vi "fpga_main.vi"() -> ()   [LabVIEW 2019]
uses:
  <vilib>/Platform/TimedLoop/XDataNode/timing_clust.ctl
  <vilib>/Platform/TimedLoop/XDataNode/nitl_modes.ctl
  <vilib>/Platform/TimedLoop/XDataNode/wakeup.ctl
  <vilib>/rvi/Emulation/niFpgaSctlEmulationGetInTimedLoop.vi
  <vilib>/rvi/Emulation/niFpgaEmulationReportErrorSimple.vi
  <vilib>/rvi/Emulation/niFpgaGetClockAttributes.vi
  <vilib>/rvi/Emulation/niFpgaCriticalErrorInLSC.vi
  <vilib>/rvi/eio/common/nirviEmuTemplateMethod_errors.vi
  <vilib>/rvi/Memory/Memory_Emulation/nirvimemoryFastEmulation.vi
  <vilib>/rvi/Memory/Memory_Emulation/nirvimemoryEmulation.vi
  <vilib>/rvi/Emulation/niFpgaEmulationIsFPGAContextNoSignature.vi
  <vilib>/rvi/DataTransferAndStorage/Container/Common/niFpgaContainerGetUniqueNameForEmu.vi
  <vilib>/rvi/Emulation/niFpgaProcessEmulError.vi
  <vilib>/rvi/errors/nirviReportUnexpectedCaseInternalError (U32).vi
  <vilib>/rvi/interface/RandomDataEmulation/niFpgaRandomDataHandleErrors.vi
  <vilib>/Platform/TimedLoop/XDataNode/XDataNode.xnode
  <vilib>/eio/EIONode/EIONode.xnode
  <vilib>/rvi/DataTransferAndStorage/Container/XNode/niFpgaContainer.xnode
  <vilib>/rvi/interface/RandomDataEmulation/nirviRandomDataFpgaReadWriteTemplate.vi
  <vilib>/Platform/TimedLoop/XDataNode/XDNodeRunTimeDep.lvlib
panel:
  in  "prog ncmd":u32
  in  "default out":u8
  in  "software trig":bool=TRUE
  in  "persistent trig":bool=TRUE
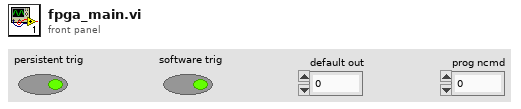
[diagram p1: front panel]
types:
  T1 = cluster{"state":enum8{"exec", "prog"}, "address":u32, "tic":u64, "init?":bool}
  T2 = typedef "XDNodeRunTimeDep.lvlib/timing_clust.ctl" = cluster{"Expected End [f-1]":u64, "Actual End [f-1]":u64, "Finished Late? [f-1]":bool, "Expected End [i-1]":u64, "Actual End [i-1]":u64, "Finished Late? [i-1]":bool, "Expected Start [i]":u64, "Actual Start [i]":u64, "Expected Start [f]":u64, "Actual Start [f]":u64, "Source Name":string, "Structure Name":string, "Period":i64, "Deadline":i64, "Offset":i64, "Start":i64, "Priority":i32, "Timeout":i32, "Mode":T3, "Wakeup Reason":T4, "Error":errorcluster, "Source Type":string, "Secondary Source Type":string, "Global End Time":u64, "Global Start Time":u64, "Frame Duration":u64, "Iteration Duration":u64, "Assigned CPU":i32, "I/O Scan Engine Mode":u32}
  T3 = typedef "XDNodeRunTimeDep.lvlib/nitl_modes.ctl" = enum32{"No Change", "Process missed periods, maintain original phase", "Discard missed periods, maintain original phase", "Process missed periods, ignore original phase", "Discard missed periods, ignore original phase"}
  T4 = typedef "XDNodeRunTimeDep.lvlib/wakeup.ctl" = enum32{"Normal", "Aborted", "Asynchronous wakeup", "Timing source error", "Timed loop error", "Timeout"}
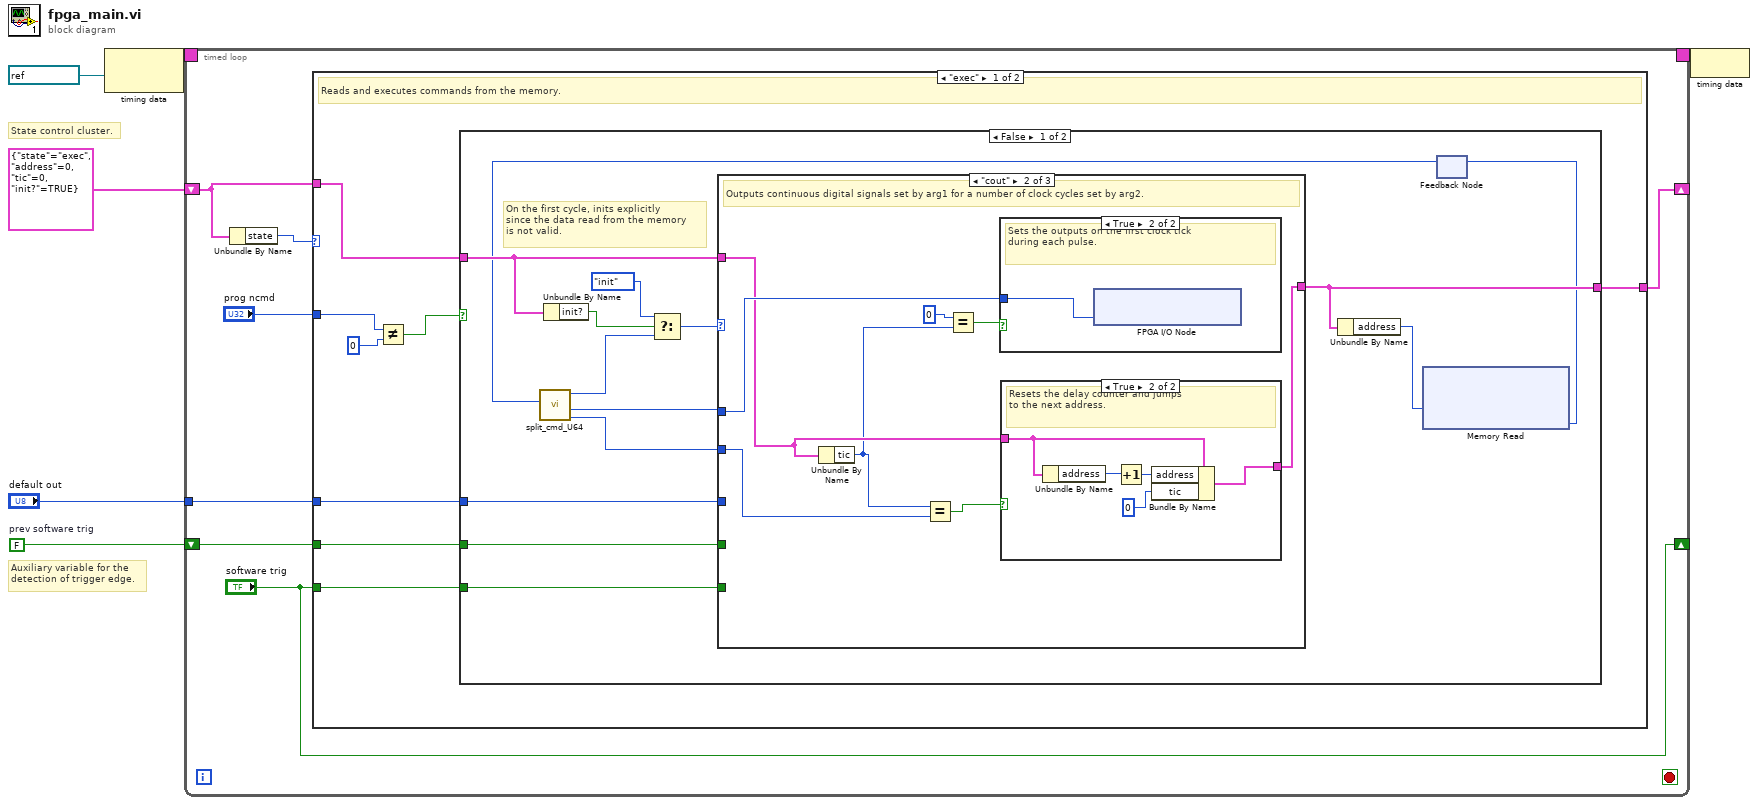
[diagram p0: block diagram]
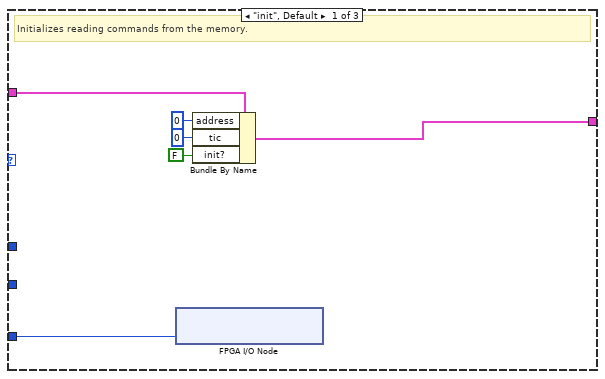
[diagram p2: hidden frame]
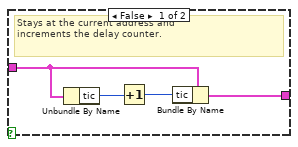
[diagram p4: hidden frame]
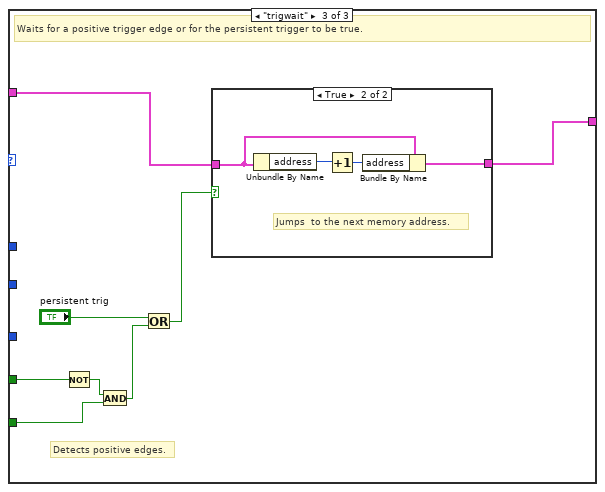
[diagram p5: hidden frame]
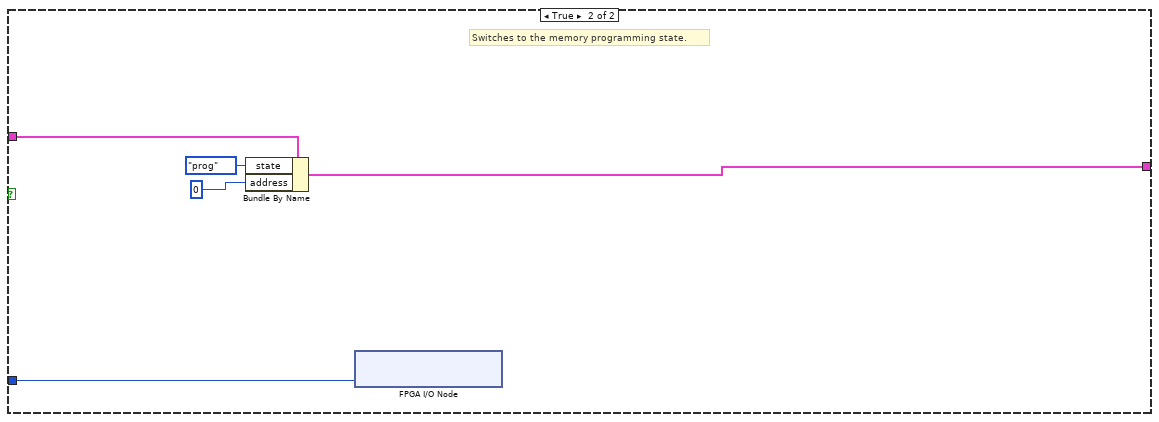
[diagram p7: hidden frame]
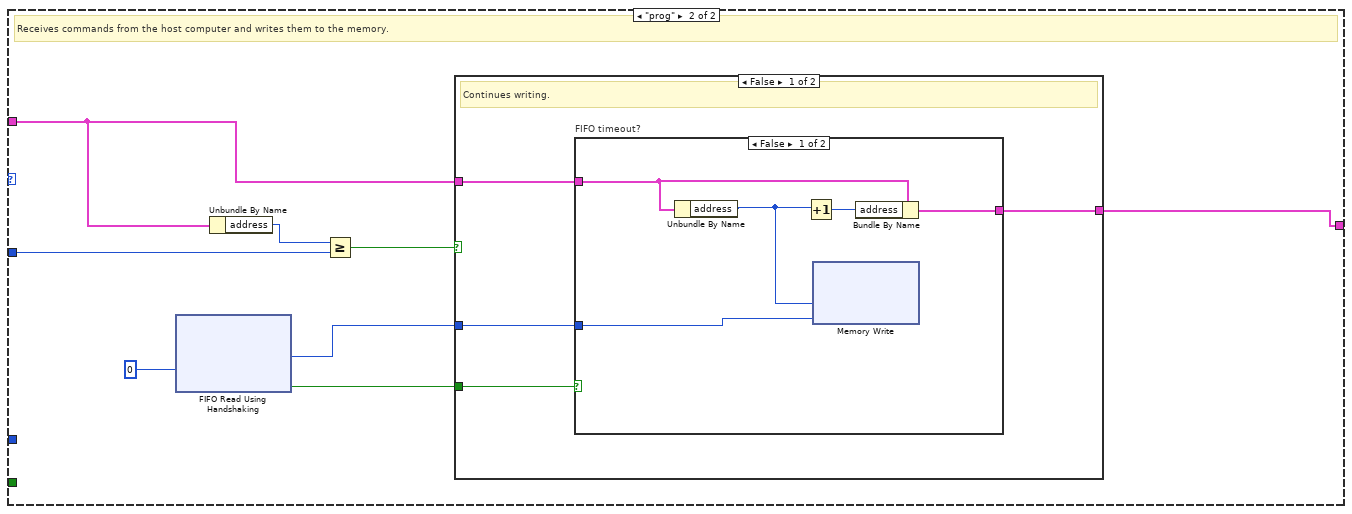
[diagram p8: hidden frame]
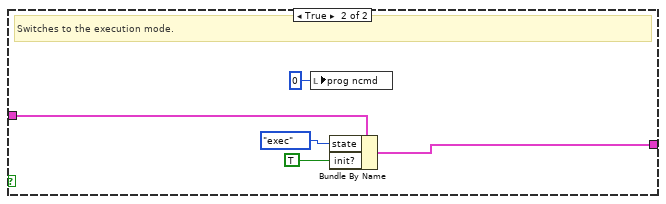
[diagram p10: hidden frame]
diagram:
  w1 = FALSE  # prev software trig
  # "Auxiliary variable for the \ndetection of trigger edge."
  # "State control cluster."
  n1 = node-c288(refnum<k21> "100MHz" ("Source Name")) -> (w6:T2)
  n2 = timed-loop {
    timing: w6 -> [_]
    timing-out: [_] -> w5
    shift-right: [w11] -> _
    shift-left: T1 {"state"=enum."exec", "address"=0, "tic"=0, "init?"=TRUE} -> [w12]
    tunnel: "default out" -> [w10]
    shift-right: ["software trig"] -> _
    shift-left: w1 -> [w9]
    stop <- _ stop-if-true
    n3 = Unbundle By Name(w12) -> ("state"=w13:enum8{"exec", "prog"})
    n4 = case shown="\"exec\"" w13 {
      tunnel: w12 -> [w21 w83]
      tunnel: [w20 w85] -> w11
      tunnel: w10 -> [w17 _]
      tunnel: w9 -> [w16 _]
      tunnel: "software trig" -> [w15 _]
      tunnel: "prog ncmd" -> [w14 w82]
      frame "exec" {
        # "Reads and executes commands from the memory."
        n5 = Not Equal?(x=w14, y=u32 0 ("x")) -> (x != y?=w19:bool)
        n6 = case shown="False" w19 {
          tunnel: w21 -> [w27 w77]
          tunnel: [w34 w76] -> w20
          tunnel: w17 -> [w35 w74]
          tunnel: w16 -> [w32 _]
          tunnel: w15 -> [w31 _]
          frame False {
            # "On the first cycle, inits explicitly \nsince the data read from the memory \nis not valid."
            n7 = Unbundle By Name(w27) -> ("init?"=w26:bool)
            n8 = feedback #1() -> (w25:u64)  [unwired: 1 in]
            n9 = call "split_cmd_U64.vi"("command"=w25) -> ("arg2"=w22:u64, "arg1"=w23:u8, "name"=w24:enum8{"init", "cout", "trigwait"})  [unwired: 7 in]
            n10 = Select(t=enum8{"init", "cout", "trigwait"}."init", s=w26, f=w24) -> (s? t:f=w29:enum8{"init", "cout", "trigwait"})
            n11 = case shown="\"cout\"" w29 {
              tunnel: w35 -> [w41 _ _]
              tunnel: [w38 w44 w65] -> w34
              tunnel: w27 -> [w40 w43 w66]
              tunnel: w23 -> [_ w46 _]
              tunnel: w32 -> [_ _ w63]
              tunnel: w31 -> [_ _ w61]
              tunnel: w22 -> [_ w45 _]
              frame "init", Default {
                # "Initializes reading commands from the memory."
                n12 = xnode "FPGA I/O Node"("ConnectorA/DIO7:0"=w41) -> ()  [unwired: 1 in, 1 out]
                n13 = Bundle By Name(cluster=w40, "address"=u32 0, "tic"=u64 0 ("tick"), "init?"=FALSE) -> (w38:T1)
              }
              frame "cout" {
                # "Outputs continuous digital signals set by arg1 for a number of clock cycles set by arg2."
                n14 = Unbundle By Name(w43) -> ("tic"=w42:u64)
                n15 = Equal?(x=w42, y=w45) -> (x = y?=w49:bool)
                n16 = Equal?(x=u64 0, y=w42) -> (x = y?=w48:bool)
                n17 = case shown="True" w48 {
                  tunnel: w46 -> [_ w50]
                  frame False {
                    # "Does nothing."
                  }
                  frame True {
                    # "Sets the outputs on the first clock tick \nduring each pulse."
                    n18 = xnode "FPGA I/O Node"("ConnectorA/DIO7:0"=w50) -> ()  [unwired: 1 in, 1 out]
                  }
                }
                n19 = case shown="True" w49 {
                  tunnel: w43 -> [w51 w59]
                  tunnel: [w53 w58] -> w44
                  frame False {
                    # "Stays at the current address and \nincrements the delay counter."
                    n20 = Unbundle By Name(w51) -> ("tic"=w52:u64)
                    n21 = Increment(x=w52) -> (x+1=w54:u64)
                    n22 = Bundle By Name(cluster=w51, "tic"=w54) -> (w53:T1)
                  }
                  frame True {
                    # "Resets the delay counter and jumps \nto the next address."
                    n23 = Unbundle By Name(w59) -> ("address"=w57:u32)
                    n24 = Increment(x=w57) -> (x+1=w56:u32)
                    n25 = Bundle By Name(cluster=w59, "address"=w56, "tic"=u64 0 ("tick")) -> (w58:T1)
                  }
                }
              }
              frame "trigwait" {
                # "Detects positive edges."
                # "Waits for a positive trigger edge or for the persistent trigger to be true."
                n26 = Not(x=w63) -> (.not. x?=w62:bool)
                n27 = And(x=w62, y=w61) -> (x .and. y?=w64:bool)
                n28 = Or(x="persistent trig", y=w64) -> (x .or. y?=w67:bool)
                n29 = case shown="True" w67 {
                  tunnel: w66 -> [w68 w72]
                  tunnel: [w68 w71] -> w65
                  frame False {
                    # "Stays at the current address."
                  }
                  frame True {
                    # "Jumps  to the next memory address."
                    n30 = Unbundle By Name(w72) -> ("address"=w70:u32)
                    n31 = Increment(x=w70) -> (x+1=w69:u32)
                    n32 = Bundle By Name(cluster=w72, "address"=w69) -> (w71:T1)
                  }
                }
              }
            }
            n33 = Unbundle By Name(w34) -> ("address"=w33:u32)
            n34 = xnode ("Memory Read")("Address"=w33) -> ("Data"=w30:u64)  [unwired: 1 in, 1 out]
            n35 = feedback-in #1(w30) -> ()
          }
          frame True {
            # "Switches to the memory programming state."
            n36 = Bundle By Name(cluster=w77, "state"=enum8{"exec", "prog"}."prog", "address"=u32 0) -> (w76:T1)
            n37 = xnode "FPGA I/O Node"("ConnectorA/DIO7:0"=w74) -> ()  [unwired: 1 in, 1 out]
          }
        }
      }
      frame "prog" {
        # "Receives commands from the host computer and writes them to the memory."
        n38 = xnode ("FIFO Read Using Handshaking")("Timeout"=0) -> ("Element"=w78:u64, "Timed Out?"=w79:bool)  [unwired: 1 in, 1 out]
        n39 = Unbundle By Name(w83) -> ("address"=w81:u32)
        n40 = Greater Or Equal?(x=w81, y=w82) -> (x >= y?=w84:bool)
        n41 = case shown="False" w84 {
          tunnel: w83 -> [w89 w97]
          tunnel: [w88 w96] -> w85
          tunnel: w79 -> [w87 _]
          tunnel: w78 -> [w86 _]
          frame False {
            # "Continues writing."
            n42 = case "FIFO timeout?" shown="False" w87 {
              tunnel: w89 -> [w91 w95]
              tunnel: [w92 w95] -> w88
              tunnel: w86 -> [w94 _]
              frame False {
                n43 = Unbundle By Name(w91) -> ("address"=w90:u32)
                n44 = Increment(x=w90) -> (x+1=w93:u32)
                n45 = xnode ("Memory Write")("Address"=w90, "Data"=w94) -> ()  [unwired: 1 in, 1 out]
                n46 = Bundle By Name(cluster=w91, "address"=w93) -> (w92:T1)
              }
              frame True {
              }
            }
          }
          frame True {
            # "Switches to the execution mode."
            n47 = local write "prog ncmd"(u32 0 ("prog ncmd")) -> ()
            n48 = Bundle By Name(cluster=w97, "state"=enum8{"exec", "prog"}."exec", "init?"=TRUE) -> (w96:T1)
          }
        }
      }
    }
  }
  n49 = node-c288(w5) -> ()
